vi "WritingDataFile Message Loop.vi"(8 "error in (no error)":errorcluster, 11 "Message Queues":T1) -> (0 "error out":errorcluster)   [LabVIEW 2020, in "WritingDataFile.lvlib"]
uses:
  WritingDataFile.lvlib
  support/Message Queue/All Message Queues.ctl
  support/Message Queue/Message Cluster.ctl
  Modbus/Modbus PLC Data All.ctl
  Modbus/Modbus FVIR Control.ctl
  Modbus/Modbus Timing.ctl
  <vilib>/Utility/miscctls.llb/LVDateTimeRec.ctl
  Modbus/Modbus LDO Control.ctl
  Data to Save.ctl
  support/Terminate Conditions Cluster.ctl
  <vilib>/Utility/file.llb/Write Delimited Spreadsheet (string).vi
  support/Message Queue/Enqueue Message (Single).vi
  support/Message Queue/Message Queue.lvlib
  Logging/Logging.lvlib
  HeaderForCSV.ctl
  HeaderForCSV_LDO.ctl
panel:
  out "Numeric":i32
  out "Loop counter":i32
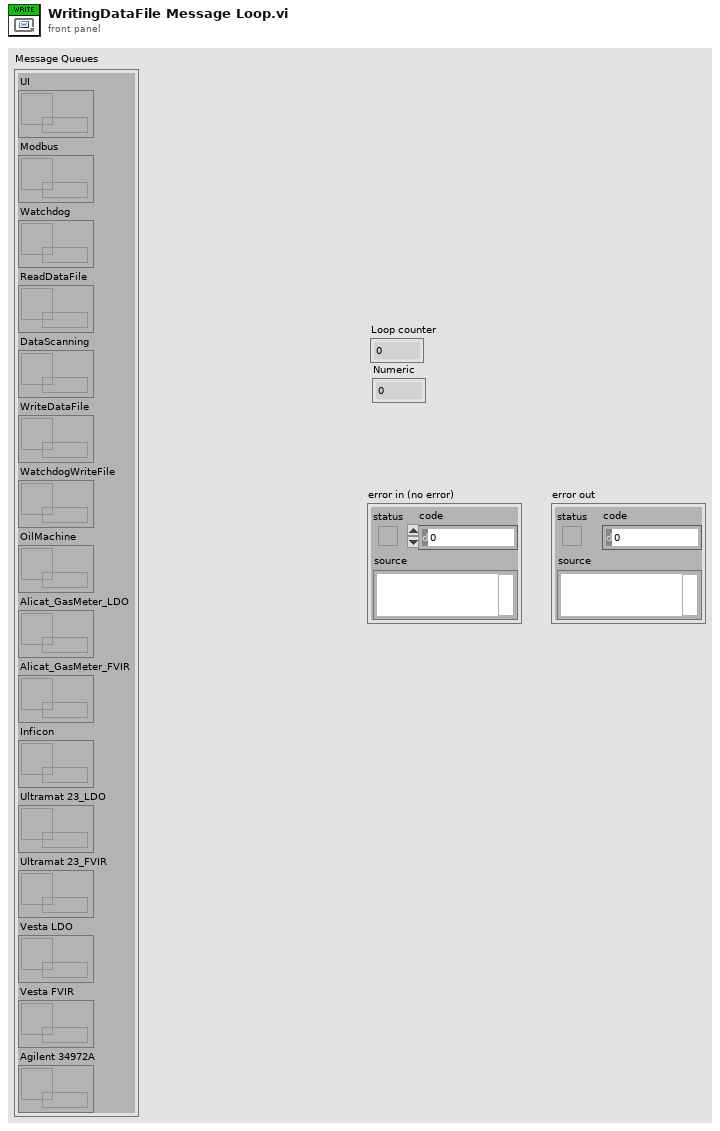
[diagram p1: front panel]
types:
  T1 = typedef "Message Queue.lvlib/All Message Queues.ctl" = cluster{"UI":refnum<queue>, "Modbus":refnum<queue>, "Watchdog":refnum<queue>, "ReadDataFile":refnum<queue>, "DataScanning":refnum<queue>, "WriteDataFile":refnum<queue>, "WatchdogWriteFile":refnum<queue>, "OilMachine":refnum<queue>, "Alicat_GasMeter_LDO":refnum<queue>, "Inficon":refnum<queue>, "Ultramat 23_LDO":refnum<queue>, "Alicat_GasMeter_FVIR":refnum<queue>, "Ultramat 23_FVIR":refnum<queue>, "Vesta LDO":refnum<queue>, "Vesta FVIR":refnum<queue>, "Agilent 34972A":refnum<queue>}
  T2 = typedef "Modbus PLC Data All.ctl" = cluster{"PLC Data - FVIR":T3, "PLC Data - LDO":T6, "PLC Registers - ALL":i16[], "Data to Save - ALL":T7, "Terminate Conditions - LDO":T8, "Terminate Conditions - FVIR":cluster{"SRI Butane Values":string[][], "Stop FVIR Test":bool}}
  T3 = typedef "Modbus FVIR Control.ctl" = cluster{"Reset FVIR Totalizer (Status)":bool, "Spare 14":bool, "Actuator mannequin is going to Work Pos - FVIR":bool, "Actuator mannequin is going to Home Pos - FVIR":bool, "Test chamber is in sequence - FVIR ":bool, "Water flow DRK375 is open - FVIR":bool, "Gas Solenoid Valve - FVIR":bool, "Water Inlet Valve - FVIR":bool, "Water Outlet Flow Proportional - FVIR":bool, "Start recording data - FVIR":bool, "Actuator spill can is going to Work Pos - FVIR":bool, "Actuator spill can is going to Home Pos - FVIR":bool, "Water Outlet Valve - FVIR":bool, "Can is spilling - FVIR":bool, "Mannequin is moving - FVIR":bool, "FVIR PLC lifebit":bool, "Status for Error - FVIR":string, "Error-FVIR":bool, "Sensor Data -FVIR":string[][], "Totalized Flow (Gallons)":dbl, "Timing":T4}
  T4 = typedef "Modbus Timing.ctl" = cluster{"First Call Time Ref":dbl, "Precondition Time Ref":dbl, "Test Time Ref":dbl, "Get First Call Time":bool, "Get Precondition Time":bool, "Get Test Time":bool, "Display Time":dbl, "Real-Time Clock":T5, "Absolute Time":dbl}
  T5 = typedef "LVDateTimeRec.ctl" = cluster{"fractional second":dbl, "second":i32, "minute":i32, "hour":i32, "day of month":i32, "month":i32, "year":i32, "day of week":i32, "day of year":i32, "DST":i32}
  T6 = typedef "Modbus LDO Control.ctl" = cluster{"LDO PLC Life Bit":bool, "Start recording data - LDO":bool, "Spare 1":bool, "Water Outlet Valve - LDO":bool, "Water Inlet Valve - LDO":bool, "Gas Solenoid Valve - LDO":bool, "Water flow DRK375 is open - LDO":bool, "Test chamber is in sequence - LDO":bool, "Oil spray 0.8cc/min - LDO":bool, "Oil spray 1.1cc/min - LDO":bool, "Oil spray 1.33cc/min - LDO":bool, "Rotary Actuator (ON/OFF) - LDO":bool, "Water Outlet Flow Proportional - LDO":bool, "Conveyor ON/OFF":bool, "Blower ON/OFF":bool, "Reset LDO Totalizer (Status)":bool, "Status for error - LDO":string, "Error - LDO":bool, "Sensor Data - LDO":string[][], "Thermal Efficiency Rate (GPM)":dbl, "Thermal Efficiency":dbl, "Totalized Flow (Gallons)":dbl, "Counter of oil injections 1.33 cc/min":u16, "Total Cycle Counter":u16, "Counter of oil injections 1.1 cc/min":u16, "Counter of oil injections 0.8 cc/min":u16, "Timing":T4}
  T7 = typedef "Data to Save.ctl" = cluster{"LDO Full Data":string[][], "FVIR Full Data":string[][], "Test Case - FVIR":string, "Test Case - LDO":string}
  T8 = typedef "Terminate Conditions Cluster.ctl" = cluster{"Condition B - Array":dbl[][], "Current Cycle":u16, "Condition C - Array":dbl[][], "Condition A - Array":dbl[][], "400 PPM Disable Counter":bool, "Condition A - Norm":dbl[][], "Condition B - Norm":dbl[][], "Condition C - Norm":dbl[][], "Condition A":bool, "Condition B":bool, "Condition C":bool, "Condition A - Cont Cycle":dbl[][], "Stop Test":bool}
  T9 = typedef "WritingDataFile.lvlib/HeaderForCSV.ctl" = string[]
  T10 = typedef "WritingDataFile.lvlib/HeaderForCSV_LDO.ctl" = string[]
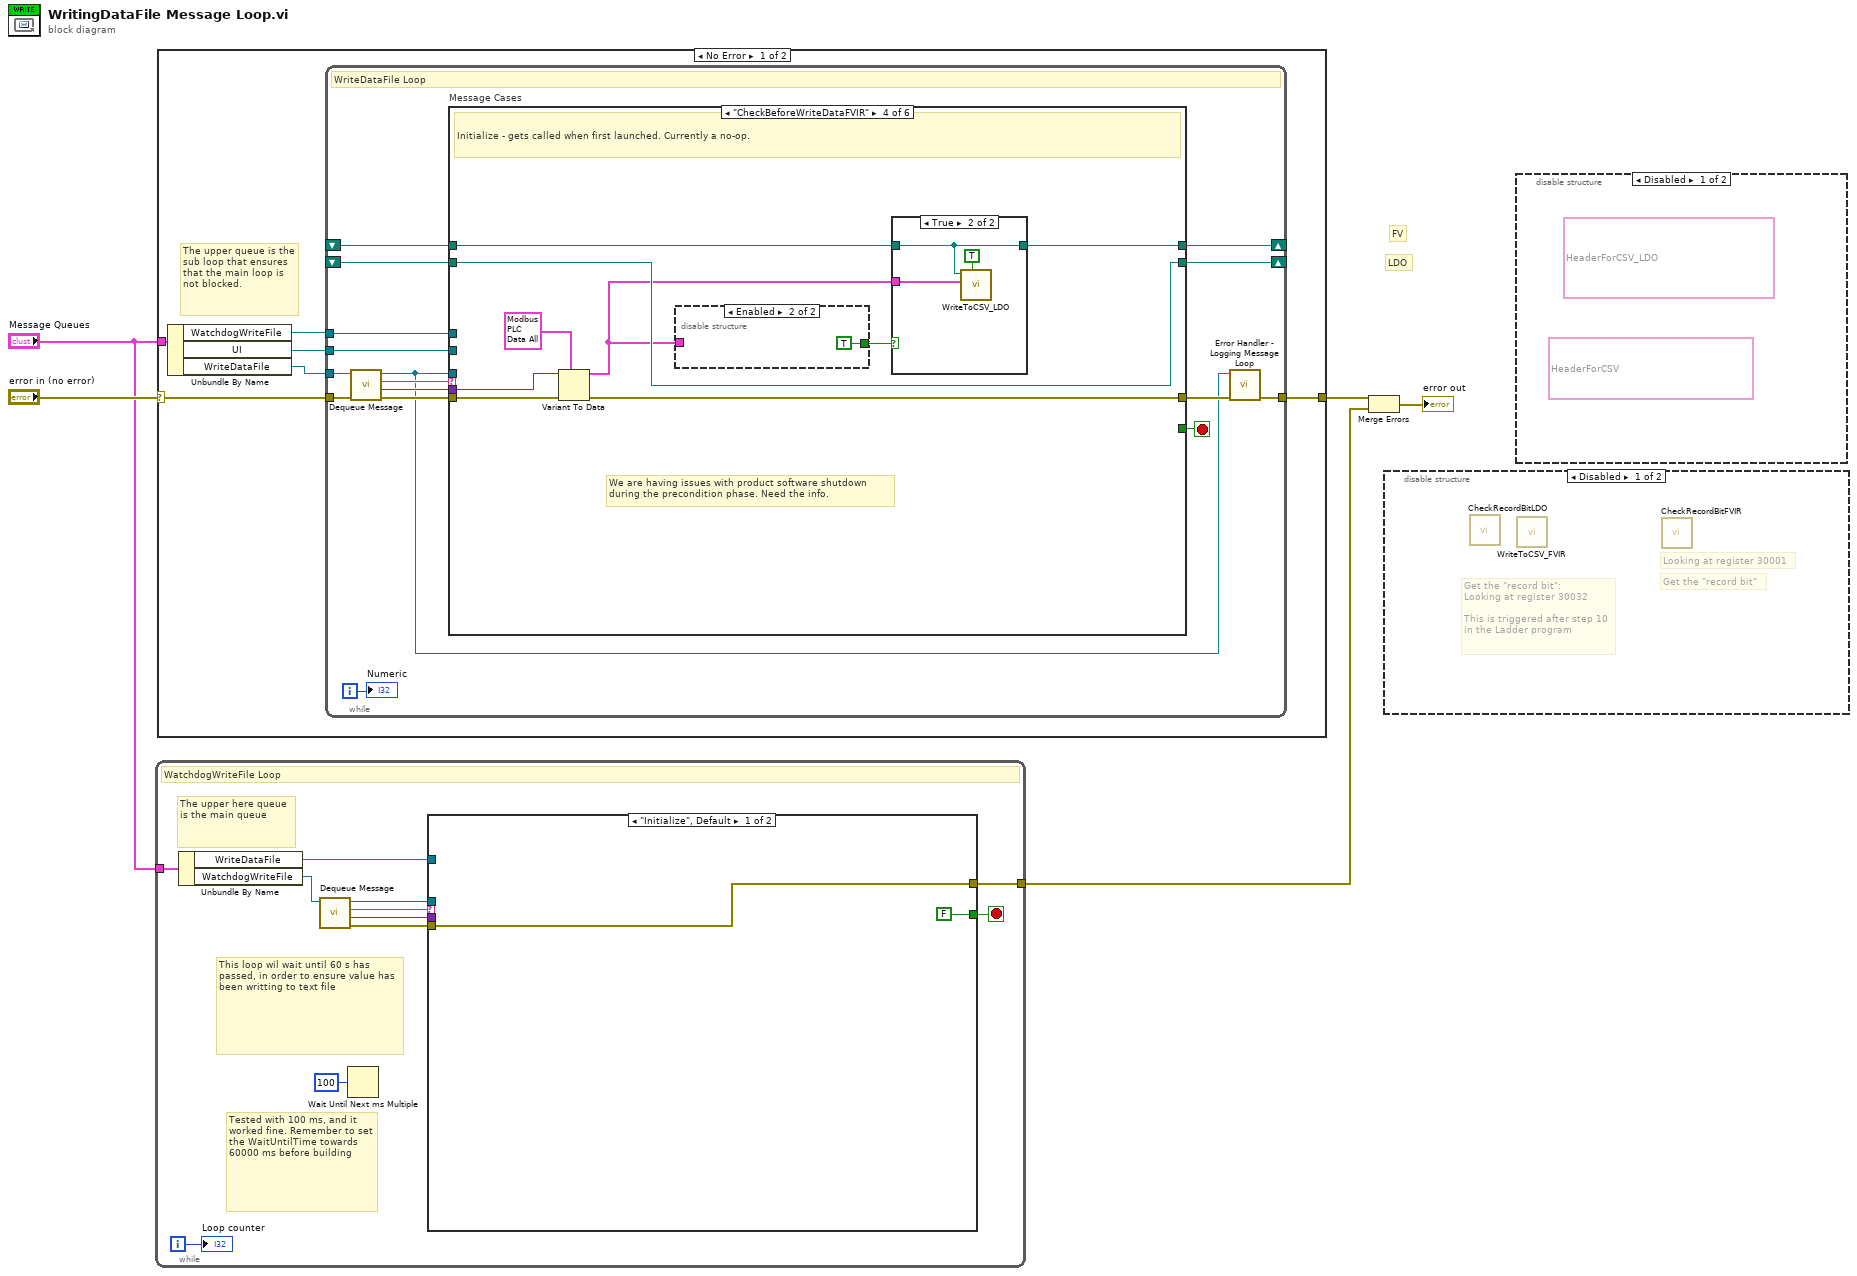
[diagram p0: block diagram]
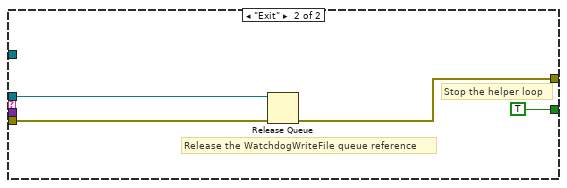
[diagram p4: hidden frame]
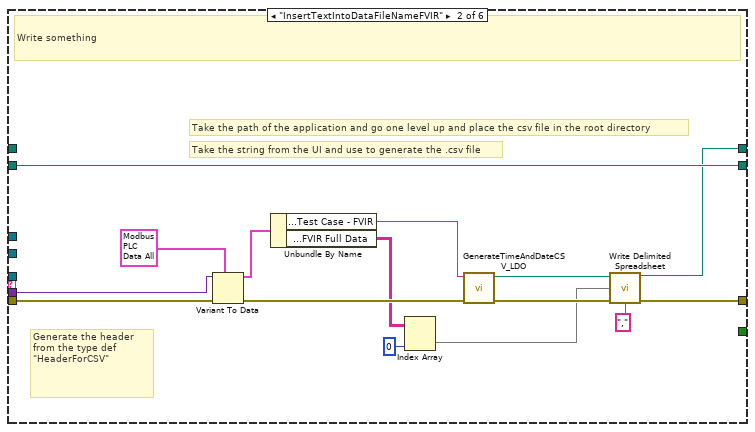
[diagram p6: hidden frame]
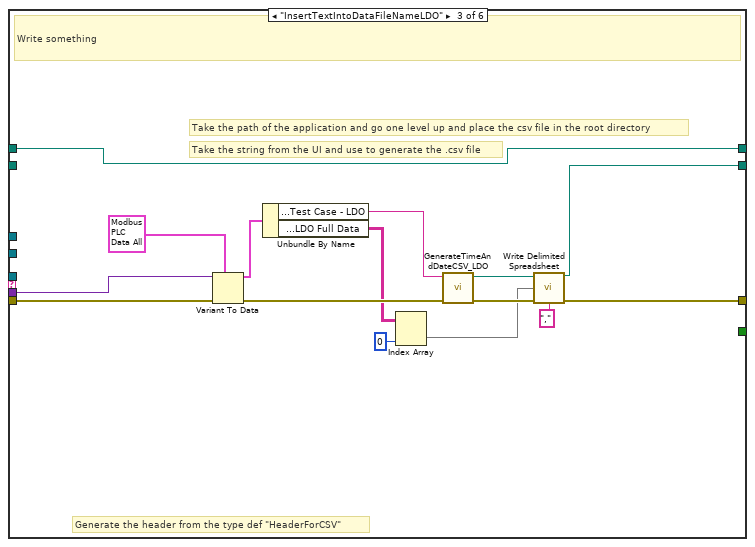
[diagram p7: hidden frame]
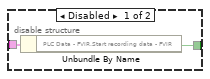
[diagram p8: hidden frame]
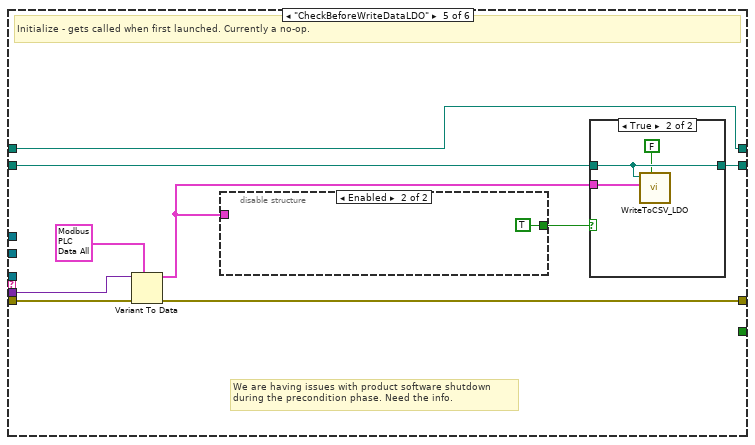
[diagram p10: hidden frame]
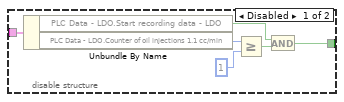
[diagram p11: hidden frame]
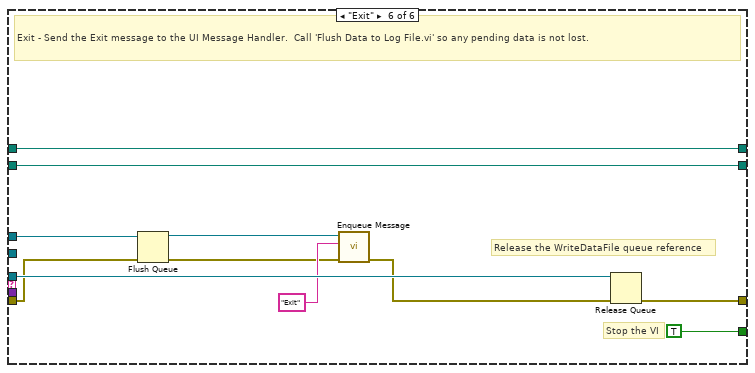
[diagram p13: hidden frame]
diagram:
  # "LDO"
  # "FV"
  n1 = while {
    tunnel: "Message Queues" -> [w16]
    tunnel: [w12] -> w2
    i -> [w7]
    stop <- w13 stop-if-true
    # "Tested with 100 ms, and it worked fine. Remember to set the WaitUntilTime towards 60000 ms before building"
    # "The upper here queue is the main queue"
    # "This loop wil wait until 60 s has passed, in order to ensure value has been writting to text file"
    # "WatchdogWriteFile Loop"
    n2 = Unbundle By Name(w16) -> ("WriteDataFile"=w10:refnum<queue>, "WatchdogWriteFile"=w11:refnum<queue>)
    n3 = call "Dequeue Message.vi"("Message Queue"=w11) -> ("error out"=w14:errorcluster, "Message Data"=w6:variant, "Message"=w15:string, "dup Message Queue"=w9:refnum<queue>)  [unwired: 7 in]
    n4 = Wait Until Next ms Multiple(millisecond multiple=u32 100) -> ()  [unwired: 1 out]
    n5 = case shown="\"Initialize\", Default" w15 {
      tunnel: w14 -> [w18 w22]
      tunnel: [w18 w21] -> w12
      tunnel: [FALSE TRUE] -> w13
      tunnel: w10 -> [_ _]
      tunnel: w9 -> [_ w19]
      tunnel: w6 -> [_ _]
      frame "Initialize", Default {
      }
      frame "Exit" {
        # "Release the WatchdogWriteFile queue reference"
        # "Stop the helper loop"
        n6 = Release Queue(queue=w19, error in (no error)=w22) -> (error out=w21:errorcluster)  [unwired: 1 in, 2 out]
      }
    }
    "Loop counter" <- w7
  }
  n7 = case shown="No Error" "error in (no error)" {
    selector: "error in (no error)" -> [w26 w125]
    tunnel: "Message Queues" -> [w28 _]
    tunnel: [w27 w125] -> w3
    frame No Error {
      # "The upper queue is the sub loop that ensures that the main loop is not blocked."
      n8 = Unbundle By Name(w28) -> ("WatchdogWriteFile"=w25:refnum<queue>, "UI"=w23:refnum<queue>, "WriteDataFile"=w24:refnum<queue>)
      n9 = while {
        tunnel: w24 -> [w39]
        tunnel: w25 -> [w36]
        tunnel: w26 -> [w43]
        tunnel: [w38] -> w27
        tunnel: w23 -> [w34]
        shift-right: [w32] -> _
        shift-left: _ -> [w31]
        shift-right: [w30] -> _
        shift-left: _ -> [w29]
        i -> [w33]
        stop <- w44 stop-if-true
        # "WriteDataFile Loop"
        n10 = call "Dequeue Message.vi"("error in (no error)"=w43, "Message Queue"=w39) -> ("error out"=w42:errorcluster, "Message Data"=w40:variant, "Message"=w41:string, "dup Message Queue"=w35:refnum<queue>)  [unwired: 6 in]
        n11 = case "Message Cases" shown="\"CheckBeforeWriteDataFVIR\"" w41 {
          tunnel: w35 -> [_ _ _ _ _ w123]
          tunnel: w42 -> [w47 w62 w77 w86 w102 w115]
          tunnel: [w47 w55 w70 w84 w100 w122] -> w37
          tunnel: [_ _ _ _ _ TRUE] -> w44
          tunnel: w40 -> [_ w61 w76 w85 w101 _]
          tunnel: w36 -> [_ _ _ _ _ w117]
          tunnel: w34 -> [_ _ _ _ _ _]
          tunnel: [w45 w60 w69 w81 w98 w118] -> w32
          tunnel: w31 -> [w45 w60 _ w81 w99 w118]
          tunnel: [w46 w54 w74 w83 w97 w119] -> w30
          tunnel: w29 -> [w46 _ w74 w82 w97 w119]
          frame "Initialize", Default {
            # "Initialize - gets called when first launched. Currently a no-op."
          }
          frame "InsertTextIntoDataFileNameFVIR" {
            # "Generate the header from the type def \"HeaderForCSV\""
            # "Take the string from the UI and use to generate the .csv file"
            # "Take the path of the application and go one level up and place the csv file in the root directory"
            # "Write something"
            n12 = Variant To Data(error in=w62, type=T2 {"PLC Data - FVIR"={"Reset FVIR Totalizer (Status)"=FALSE, "Spare 14"=FALSE, "Actuator mannequin is going to Work Pos - FVIR"=FALSE, "Actuator mannequin is going to Home Pos - FVIR"=FALSE, "Test chamber is in sequence - FVIR "=FALSE, "Water flow DRK375 is open - FVIR"=FALSE, "Gas Solenoid Valve - FVIR"=FALSE, "Water Inlet Valve - FVIR"=FALSE, "Water Outlet Flow Proportional - FVIR"=FALSE, "Start recording data - FVIR"=FALSE, "Actuator spill can is going to Work Pos - FVIR"=FALSE, "Actuator spill can is going to Home Pos - FVIR"=FALSE, "Water Outlet Valve - FVIR"=FALSE, "Can is spilling - FVIR"=FALSE, "Mannequin is moving - FVIR"=FALSE, "FVIR PLC lifebit"=FALSE, "Status for Error - FVIR"="", "Error-FVIR"=FALSE, "Sensor Data -FVIR"=[], "Totalized Flow (Gallons)"=0.0, "Timing"={"First Call Time Ref"=0.0, "Precondition Time Ref"=0.0, "Test Time Ref"=0.0, "Get First Call Time"=FALSE, "Get Precondition Time"=FALSE, "Get Test Time"=FALSE, "Display Time"=0.0, "Real-Time Clock"={"fractional second"=0.0, "second"=0, "minute"=0, "hour"=0, "day of month"=0, "month"=0, "year"=0, "day of week"=0, "day of year"=0, "DST"=0}, "Absolute Time"=0.0}}, "PLC Data - LDO"={"LDO PLC Life Bit"=FALSE, "Start recording data - LDO"=FALSE, "Spare 1"=FALSE, "Water Outlet Valve - LDO"=FALSE, "Water Inlet Valve - LDO"=FALSE, "Gas Solenoid Valve - LDO"=FALSE, "Water flow DRK375 is open - LDO"=FALSE, "Test chamber is in sequence - LDO"=FALSE, "Oil spray 0.8cc/min - LDO"=FALSE, "Oil spray 1.1cc/min - LDO"=FALSE, "Oil spray 1.33cc/min - LDO"=FALSE, "Rotary Actuator (ON/OFF) - LDO"=FALSE, "Water Outlet Flow Proportional - LDO"=FALSE, "Conveyor ON/OFF"=FALSE, "Blower ON/OFF"=FALSE, "Reset LDO Totalizer (Status)"=FALSE, "Status for error - LDO"="", "Error - LDO"=FALSE, "Sensor Data - LDO"=[], "Thermal Efficiency Rate (GPM)"=0.0, "Thermal Efficiency"=0.0, "Totalized Flow (Gallons)"=0.0, "Counter of oil injections 1.33 cc/min"=0, "Total Cycle Counter"=0, "Counter of oil injections 1.1 cc/min"=0, "Counter of oil injections 0.8 cc/min"=0, "Timing"={"First Call Time Ref"=0.0, "Precondition Time Ref"=0.0, "Test Time Ref"=0.0, "Get First Call Time"=FALSE, "Get Precondition Time"=FALSE, "Get Test Time"=FALSE, "Display Time"=0.0, "Real-Time Clock"={"fractional second"=0.0, "second"=0, "minute"=0, "hour"=0, "day of month"=0, "month"=0, "year"=0, "day of week"=0, "day of year"=0, "DST"=0}, "Absolute Time"=0.0}}, "PLC Registers - ALL"=[], "Data to Save - ALL"={"LDO Full Data"=[], "FVIR Full Data"=[], "Test Case - FVIR"="", "Test Case - LDO"=""}, "Terminate Conditions - LDO"={"Condition B - Array"=[], "Current Cycle"=0, "Condition C - Array"=[], "Condition A - Array"=[], "400 PPM Disable Counter"=FALSE, "Condition A - Norm"=[], "Condition B - Norm"=[], "Condition C - Norm"=[], "Condition A"=FALSE, "Condition B"=FALSE, "Condition C"=FALSE, "Condition A - Cont Cycle"=[], "Stop Test"=FALSE}, "Terminate Conditions - FVIR"={"SRI Butane Values"=[], "Stop FVIR Test"=FALSE}} ("PLC Data Out"), Variant=w61) -> (data=w53:T2, error out=w58:errorcluster)
            n13 = Unbundle By Name(w53) -> ("Data to Save - ALL.Test Case - FVIR"=w52:string, "Data to Save - ALL.FVIR Full Data"=w50:string[][])
            n14 = Index Array(array=w50, index (col)=0 ("disabled index (col)")) -> (element=w48:string[])  [unwired: 1 in]
            n15 = call "GenerateTimeAndDateCSV_LDO.vi"("error in (no error)"=w58, "Test string input"=w52) -> ("error out"=w56:errorcluster, "path for csv file"=w57:path)  [unwired: 8 in]
            n16 = call-poly <vilib>:"Write Delimited Spreadsheet.vi"("file path (dialog if empty)"=w57, "1D data"=w48, "error in (no error)"=w56, "delimiter (\\t)"="," ("delimiter (\\t)")) -> ("new file path (Not A Path if cancelled)"=w54:path, "error out"=w55:errorcluster)  [unwired: 10 in]
          }
          frame "InsertTextIntoDataFileNameLDO" {
            # "Generate the header from the type def \"HeaderForCSV\""
            # "Take the string from the UI and use to generate the .csv file"
            # "Take the path of the application and go one level up and place the csv file in the root directory"
            # "Write something"
            n17 = Variant To Data(error in=w77, type=T2 {"PLC Data - FVIR"={"Reset FVIR Totalizer (Status)"=FALSE, "Spare 14"=FALSE, "Actuator mannequin is going to Work Pos - FVIR"=FALSE, "Actuator mannequin is going to Home Pos - FVIR"=FALSE, "Test chamber is in sequence - FVIR "=FALSE, "Water flow DRK375 is open - FVIR"=FALSE, "Gas Solenoid Valve - FVIR"=FALSE, "Water Inlet Valve - FVIR"=FALSE, "Water Outlet Flow Proportional - FVIR"=FALSE, "Start recording data - FVIR"=FALSE, "Actuator spill can is going to Work Pos - FVIR"=FALSE, "Actuator spill can is going to Home Pos - FVIR"=FALSE, "Water Outlet Valve - FVIR"=FALSE, "Can is spilling - FVIR"=FALSE, "Mannequin is moving - FVIR"=FALSE, "FVIR PLC lifebit"=FALSE, "Status for Error - FVIR"="", "Error-FVIR"=FALSE, "Sensor Data -FVIR"=[], "Totalized Flow (Gallons)"=0.0, "Timing"={"First Call Time Ref"=0.0, "Precondition Time Ref"=0.0, "Test Time Ref"=0.0, "Get First Call Time"=FALSE, "Get Precondition Time"=FALSE, "Get Test Time"=FALSE, "Display Time"=0.0, "Real-Time Clock"={"fractional second"=0.0, "second"=0, "minute"=0, "hour"=0, "day of month"=0, "month"=0, "year"=0, "day of week"=0, "day of year"=0, "DST"=0}, "Absolute Time"=0.0}}, "PLC Data - LDO"={"LDO PLC Life Bit"=FALSE, "Start recording data - LDO"=FALSE, "Spare 1"=FALSE, "Water Outlet Valve - LDO"=FALSE, "Water Inlet Valve - LDO"=FALSE, "Gas Solenoid Valve - LDO"=FALSE, "Water flow DRK375 is open - LDO"=FALSE, "Test chamber is in sequence - LDO"=FALSE, "Oil spray 0.8cc/min - LDO"=FALSE, "Oil spray 1.1cc/min - LDO"=FALSE, "Oil spray 1.33cc/min - LDO"=FALSE, "Rotary Actuator (ON/OFF) - LDO"=FALSE, "Water Outlet Flow Proportional - LDO"=FALSE, "Conveyor ON/OFF"=FALSE, "Blower ON/OFF"=FALSE, "Reset LDO Totalizer (Status)"=FALSE, "Status for error - LDO"="", "Error - LDO"=FALSE, "Sensor Data - LDO"=[], "Thermal Efficiency Rate (GPM)"=0.0, "Thermal Efficiency"=0.0, "Totalized Flow (Gallons)"=0.0, "Counter of oil injections 1.33 cc/min"=0, "Total Cycle Counter"=0, "Counter of oil injections 1.1 cc/min"=0, "Counter of oil injections 0.8 cc/min"=0, "Timing"={"First Call Time Ref"=0.0, "Precondition Time Ref"=0.0, "Test Time Ref"=0.0, "Get First Call Time"=FALSE, "Get Precondition Time"=FALSE, "Get Test Time"=FALSE, "Display Time"=0.0, "Real-Time Clock"={"fractional second"=0.0, "second"=0, "minute"=0, "hour"=0, "day of month"=0, "month"=0, "year"=0, "day of week"=0, "day of year"=0, "DST"=0}, "Absolute Time"=0.0}}, "PLC Registers - ALL"=[], "Data to Save - ALL"={"LDO Full Data"=[], "FVIR Full Data"=[], "Test Case - FVIR"="", "Test Case - LDO"=""}, "Terminate Conditions - LDO"={"Condition B - Array"=[], "Current Cycle"=0, "Condition C - Array"=[], "Condition A - Array"=[], "400 PPM Disable Counter"=FALSE, "Condition A - Norm"=[], "Condition B - Norm"=[], "Condition C - Norm"=[], "Condition A"=FALSE, "Condition B"=FALSE, "Condition C"=FALSE, "Condition A - Cont Cycle"=[], "Stop Test"=FALSE}, "Terminate Conditions - FVIR"={"SRI Butane Values"=[], "Stop FVIR Test"=FALSE}} ("PLC Data Out"), Variant=w76) -> (data=w68:T2, error out=w72:errorcluster)
            n18 = Unbundle By Name(w68) -> ("Data to Save - ALL.Test Case - LDO"=w67:string, "Data to Save - ALL.LDO Full Data"=w66:string[][])
            n19 = Index Array(array=w66, index (col)=0 ("disabled index (col)")) -> (element=w63:string[])  [unwired: 1 in]
            n20 = call "GenerateTimeAndDateCSV_LDO.vi"("error in (no error)"=w72, "Test string input"=w67) -> ("error out"=w71:errorcluster, "path for csv file"=w75:path)  [unwired: 8 in]
            n21 = call-poly <vilib>:"Write Delimited Spreadsheet.vi"("file path (dialog if empty)"=w75, "1D data"=w63, "error in (no error)"=w71, "delimiter (\\t)"="," ("delimiter (\\t)")) -> ("new file path (Not A Path if cancelled)"=w69:path, "error out"=w70:errorcluster)  [unwired: 10 in]
          }
          frame "CheckBeforeWriteDataFVIR" {
            # "We are having issues with product software shutdown\nduring the precondition phase. Need the info."
            # "Initialize - gets called when first launched. Currently a no-op."
            n22 = Variant To Data(error in=w86, type=T2 {"PLC Data - FVIR"={"Reset FVIR Totalizer (Status)"=FALSE, "Spare 14"=FALSE, "Actuator mannequin is going to Work Pos - FVIR"=FALSE, "Actuator mannequin is going to Home Pos - FVIR"=FALSE, "Test chamber is in sequence - FVIR "=FALSE, "Water flow DRK375 is open - FVIR"=FALSE, "Gas Solenoid Valve - FVIR"=FALSE, "Water Inlet Valve - FVIR"=FALSE, "Water Outlet Flow Proportional - FVIR"=FALSE, "Start recording data - FVIR"=FALSE, "Actuator spill can is going to Work Pos - FVIR"=FALSE, "Actuator spill can is going to Home Pos - FVIR"=FALSE, "Water Outlet Valve - FVIR"=FALSE, "Can is spilling - FVIR"=FALSE, "Mannequin is moving - FVIR"=FALSE, "FVIR PLC lifebit"=FALSE, "Status for Error - FVIR"="", "Error-FVIR"=FALSE, "Sensor Data -FVIR"=[], "Totalized Flow (Gallons)"=0.0, "Timing"={"First Call Time Ref"=0.0, "Precondition Time Ref"=0.0, "Test Time Ref"=0.0, "Get First Call Time"=FALSE, "Get Precondition Time"=FALSE, "Get Test Time"=FALSE, "Display Time"=0.0, "Real-Time Clock"={"fractional second"=0.0, "second"=0, "minute"=0, "hour"=0, "day of month"=0, "month"=0, "year"=0, "day of week"=0, "day of year"=0, "DST"=0}, "Absolute Time"=0.0}}, "PLC Data - LDO"={"LDO PLC Life Bit"=FALSE, "Start recording data - LDO"=FALSE, "Spare 1"=FALSE, "Water Outlet Valve - LDO"=FALSE, "Water Inlet Valve - LDO"=FALSE, "Gas Solenoid Valve - LDO"=FALSE, "Water flow DRK375 is open - LDO"=FALSE, "Test chamber is in sequence - LDO"=FALSE, "Oil spray 0.8cc/min - LDO"=FALSE, "Oil spray 1.1cc/min - LDO"=FALSE, "Oil spray 1.33cc/min - LDO"=FALSE, "Rotary Actuator (ON/OFF) - LDO"=FALSE, "Water Outlet Flow Proportional - LDO"=FALSE, "Conveyor ON/OFF"=FALSE, "Blower ON/OFF"=FALSE, "Reset LDO Totalizer (Status)"=FALSE, "Status for error - LDO"="", "Error - LDO"=FALSE, "Sensor Data - LDO"=[], "Thermal Efficiency Rate (GPM)"=0.0, "Thermal Efficiency"=0.0, "Totalized Flow (Gallons)"=0.0, "Counter of oil injections 1.33 cc/min"=0, "Total Cycle Counter"=0, "Counter of oil injections 1.1 cc/min"=0, "Counter of oil injections 0.8 cc/min"=0, "Timing"={"First Call Time Ref"=0.0, "Precondition Time Ref"=0.0, "Test Time Ref"=0.0, "Get First Call Time"=FALSE, "Get Precondition Time"=FALSE, "Get Test Time"=FALSE, "Display Time"=0.0, "Real-Time Clock"={"fractional second"=0.0, "second"=0, "minute"=0, "hour"=0, "day of month"=0, "month"=0, "year"=0, "day of week"=0, "day of year"=0, "DST"=0}, "Absolute Time"=0.0}}, "PLC Registers - ALL"=[], "Data to Save - ALL"={"LDO Full Data"=[], "FVIR Full Data"=[], "Test Case - FVIR"="", "Test Case - LDO"=""}, "Terminate Conditions - LDO"={"Condition B - Array"=[], "Current Cycle"=0, "Condition C - Array"=[], "Condition A - Array"=[], "400 PPM Disable Counter"=FALSE, "Condition A - Norm"=[], "Condition B - Norm"=[], "Condition C - Norm"=[], "Condition A"=FALSE, "Condition B"=FALSE, "Condition C"=FALSE, "Condition A - Cont Cycle"=[], "Stop Test"=FALSE}, "Terminate Conditions - FVIR"={"SRI Butane Values"=[], "Stop FVIR Test"=FALSE}} ("PLC Data Out"), Variant=w85) -> (data=w79:T2, error out=w84:errorcluster)
            n23 = disable-structure shown="Enabled" {
              disable-tunnel: w79 -> [w88 _]
              disable-tunnel: [w87 TRUE ("Start recording data - FVIR")] -> w78
              frame Disabled {
                n24 = Unbundle By Name(w88) -> ("PLC Data - FVIR.Start recording data - FVIR"=w87:bool)
              }
              frame Enabled {
              }
            }
            n25 = case shown="True" w78 {
              tunnel: w79 -> [_ w93]
              tunnel: [w90 w92] -> w83
              tunnel: w82 -> [w90 w92]
              frame False {
              }
              frame True {
                n26 = call "WriteToCSV_LDO.vi"("FVIR?"=TRUE, "PLC Data Out"=w93, "file path (dialog if empty)"=w92) -> ()  [unwired: 9 in]
              }
            }
          }
          frame "CheckBeforeWriteDataLDO" {
            # "We are having issues with product software shutdown\nduring the precondition phase. Need the info."
            # "Initialize - gets called when first launched. Currently a no-op."
            n27 = Variant To Data(error in=w102, type=T2 {"PLC Data - FVIR"={"Reset FVIR Totalizer (Status)"=FALSE, "Spare 14"=FALSE, "Actuator mannequin is going to Work Pos - FVIR"=FALSE, "Actuator mannequin is going to Home Pos - FVIR"=FALSE, "Test chamber is in sequence - FVIR "=FALSE, "Water flow DRK375 is open - FVIR"=FALSE, "Gas Solenoid Valve - FVIR"=FALSE, "Water Inlet Valve - FVIR"=FALSE, "Water Outlet Flow Proportional - FVIR"=FALSE, "Start recording data - FVIR"=FALSE, "Actuator spill can is going to Work Pos - FVIR"=FALSE, "Actuator spill can is going to Home Pos - FVIR"=FALSE, "Water Outlet Valve - FVIR"=FALSE, "Can is spilling - FVIR"=FALSE, "Mannequin is moving - FVIR"=FALSE, "FVIR PLC lifebit"=FALSE, "Status for Error - FVIR"="", "Error-FVIR"=FALSE, "Sensor Data -FVIR"=[], "Totalized Flow (Gallons)"=0.0, "Timing"={"First Call Time Ref"=0.0, "Precondition Time Ref"=0.0, "Test Time Ref"=0.0, "Get First Call Time"=FALSE, "Get Precondition Time"=FALSE, "Get Test Time"=FALSE, "Display Time"=0.0, "Real-Time Clock"={"fractional second"=0.0, "second"=0, "minute"=0, "hour"=0, "day of month"=0, "month"=0, "year"=0, "day of week"=0, "day of year"=0, "DST"=0}, "Absolute Time"=0.0}}, "PLC Data - LDO"={"LDO PLC Life Bit"=FALSE, "Start recording data - LDO"=FALSE, "Spare 1"=FALSE, "Water Outlet Valve - LDO"=FALSE, "Water Inlet Valve - LDO"=FALSE, "Gas Solenoid Valve - LDO"=FALSE, "Water flow DRK375 is open - LDO"=FALSE, "Test chamber is in sequence - LDO"=FALSE, "Oil spray 0.8cc/min - LDO"=FALSE, "Oil spray 1.1cc/min - LDO"=FALSE, "Oil spray 1.33cc/min - LDO"=FALSE, "Rotary Actuator (ON/OFF) - LDO"=FALSE, "Water Outlet Flow Proportional - LDO"=FALSE, "Conveyor ON/OFF"=FALSE, "Blower ON/OFF"=FALSE, "Reset LDO Totalizer (Status)"=FALSE, "Status for error - LDO"="", "Error - LDO"=FALSE, "Sensor Data - LDO"=[], "Thermal Efficiency Rate (GPM)"=0.0, "Thermal Efficiency"=0.0, "Totalized Flow (Gallons)"=0.0, "Counter of oil injections 1.33 cc/min"=0, "Total Cycle Counter"=0, "Counter of oil injections 1.1 cc/min"=0, "Counter of oil injections 0.8 cc/min"=0, "Timing"={"First Call Time Ref"=0.0, "Precondition Time Ref"=0.0, "Test Time Ref"=0.0, "Get First Call Time"=FALSE, "Get Precondition Time"=FALSE, "Get Test Time"=FALSE, "Display Time"=0.0, "Real-Time Clock"={"fractional second"=0.0, "second"=0, "minute"=0, "hour"=0, "day of month"=0, "month"=0, "year"=0, "day of week"=0, "day of year"=0, "DST"=0}, "Absolute Time"=0.0}}, "PLC Registers - ALL"=[], "Data to Save - ALL"={"LDO Full Data"=[], "FVIR Full Data"=[], "Test Case - FVIR"="", "Test Case - LDO"=""}, "Terminate Conditions - LDO"={"Condition B - Array"=[], "Current Cycle"=0, "Condition C - Array"=[], "Condition A - Array"=[], "400 PPM Disable Counter"=FALSE, "Condition A - Norm"=[], "Condition B - Norm"=[], "Condition C - Norm"=[], "Condition A"=FALSE, "Condition B"=FALSE, "Condition C"=FALSE, "Condition A - Cont Cycle"=[], "Stop Test"=FALSE}, "Terminate Conditions - FVIR"={"SRI Butane Values"=[], "Stop FVIR Test"=FALSE}} ("PLC Data Out"), Variant=w101) -> (data=w95:T2, error out=w100:errorcluster)
            n28 = disable-structure shown="Enabled" {
              disable-tunnel: w95 -> [w108 _]
              disable-tunnel: [w103 TRUE] -> w94
              frame Disabled {
                n29 = Unbundle By Name(w108) -> ("PLC Data - LDO.Start recording data - LDO"=w104:bool, "PLC Data - LDO.Counter of oil injections 1.1 cc/min"=w107:u16)
                n30 = Greater Or Equal?(x=w107, y=u16 1) -> (x >= y?=w105:bool)
                n31 = And(x=w104, y=w105) -> (x .and. y?=w103:bool)
              }
              frame Enabled {
              }
            }
            n32 = case shown="True" w94 {
              tunnel: w95 -> [_ w112]
              tunnel: w99 -> [w110 w113]
              tunnel: [w110 w113] -> w98
              frame False {
              }
              frame True {
                n33 = call "WriteToCSV_LDO.vi"("FVIR?"=FALSE, "PLC Data Out"=w112, "file path (dialog if empty)"=w113) -> ()  [unwired: 9 in]
              }
            }
          }
          frame "Exit" {
            # "Release the WriteDataFile queue reference"
            # "Stop the VI"
            # "Exit - Send the Exit message to the UI Message Handler.  Call 'Flush Data to Log File.vi' so any pending data is not lost."
            n34 = Flush Queue(queue=w117, error in (no error)=w115) -> (queue out=w116:refnum<queue>, error out=w114:errorcluster)  [unwired: 1 out]
            n35 = call-poly "Enqueue Message.vi"("error in (no error)"=w114, "Message"="Exit", "Message Queue"=w116) -> ("error out"=w120:errorcluster)  [unwired: 7 in, 1 out]
            n36 = Release Queue(queue=w123, error in (no error)=w120) -> (error out=w122:errorcluster)  [unwired: 1 in, 2 out]
          }
        }
        n37 = call "Error Handler - Logging Message Loop.vi"("error in (no error)"=w37, "Message Queue"=w35) -> ("dup error in"=w38:errorcluster)  [unwired: 8 in, 1 out]
        "Numeric" <- w33
      }
    }
    frame Error {
    }
  }
  n38 = Merge Errors(w3, w2) -> (→"error out":errorcluster)
  n39 = disable-structure shown="Disabled" {
    frame Disabled {
      # "Looking at register 30001"
      # "Get the \"record bit\""
      # "Get the \"record bit\":\nLooking at register 30032\n\nThis is triggered after step 10\nin the Ladder program"
      n40 = call "CheckRecordBitLDO.vi"() -> ()  [unwired: 11 in, 1 out]
      n41 = call "WriteToCSV_FVIR.vi"() -> ()  [unwired: 12 in]
      n42 = call "CheckRecordBitFVIR.vi"() -> ()  [unwired: 11 in, 1 out]
    }
    frame Enabled {
    }
  }
  n43 = disable-structure shown="Disabled" {
    frame Disabled {
      (unwired) T9 ["Sample date", "Timestamp", "Starting time time", "Elapsed time seconds", "Register 30001", "Register 30002", "Register 30003", "Register 30004", "Register 30005", "Register 30006", "Register 30007", "Register 30008", "Register 30009", "Register 30010", "Register 30011", "Register 30012", "Register 30013", "Register 30014", "Register 30015", "Register 30016", "Register 30017", "Register 30018", "Register 30019", "Register 30020", "Register 30021", "Register 30022", "Register 30023", "Register 30024", "Register 30025", "Register 30026", "Register 30027", "Register 30028", "Register 30029", "Register 30030", "Register 30031"] ("new element/subarray 2")
      (unwired) T10 ["Sample date", "Timestamp", "Starting time time", "Elapsed time seconds", "Register 30032", "Register 30033", "Register 30034", "Register 30035", "Register 30036", "Register 30037", "Register 30038", "Register 30039", "Register 30040", "Register 30041", "Register 30042", "Register 30043", "Register 30044", "Register 30045", "Register 30046", "Register 30047", "Register 30048", "Register 30049", "Register 30050", "Register 30051", "Register 30052", "Register 30053", "Register 30054", "Register 30055", "Register 30056", "Register 30057"] ("new element/subarray")
    }
    frame Enabled {
    }
  }
